vi "Do.vi"(8 "error in (no error)":errorcluster, 10 "Actor in":refnum<class "Actor.lvclass">, 11 "LogStatementMsg":refnum<class "LogStatementMsg.lvclass">) -> (0 "error out":errorcluster, 2 "Actor out":refnum<class "Actor.lvclass">)   [LabVIEW 2026, in "Lumberjack.lvlib" / "LogStatementMsg.lvclass"]
doc: "<p>(<strong>Filename</strong>: <span class=\"dnl\">Actor Framework.lvlib:Message.lvclass:Do.vi</span>)</p>\n<p>Defines what a message does when it is received by an actor. Generally, a message instructs an actor to invoke one of its methods. By default, this method does nothing. A child class must override it to define behavior.</p>"
uses:
  LogStatementMsg.lvclass
  <vilib>/ActorFramework/Actor/Actor.lvclass
  Appenders/Appender.lvclass/Appender.lvclass
  LogStatementMsg.lvclass/LogStatementMsg.ctl
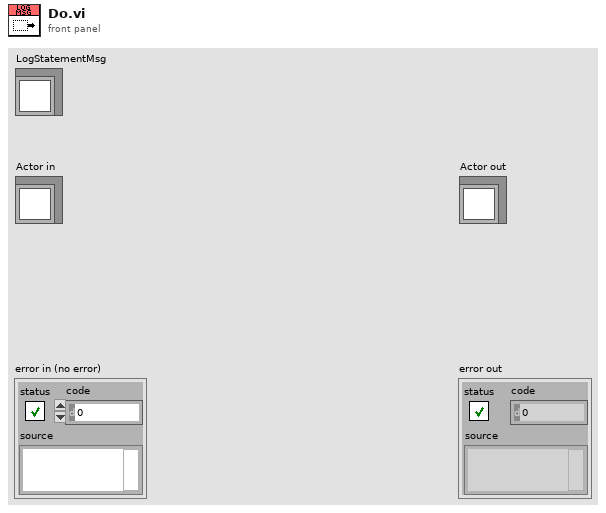
[diagram p1: front panel]
types:
  T1 = typedef "Lumberjack.lvlib/Statement.ctl" = cluster{"timestamp":timestamp, "level":T2, "sourceTag":string, "originVI":string, "message":string}
  T2 = typedef "Lumberjack.lvlib/Severity.ctl" = enum16{"OFF", "FATAL", "ERROR", "WARN", "INFO", "DEBUG", "TRACE", "ALL"}
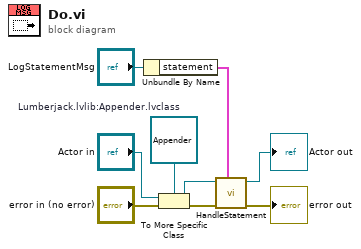
[diagram p0: block diagram]
diagram:
  w1 = refnum<class "Appender.lvclass"> refnum  # Lumberjack.lvlib:Appender.lvclass
  n1 = Unbundle By Name("LogStatementMsg") -> ("statement"=w7:T1)
  n2 = To More Specific Class(target class=w1, reference="Actor in", error in="error in (no error)") -> (specific class reference=w9:refnum<class "Appender.lvclass">, error out=w6:errorcluster)
  n3 = call "HandleStatement.vi"("Statement"=w7, "error in (no error)"=w6, "Appender in"=w9) -> ("error out"=→"error out":errorcluster, "Appender out"=→"Actor out":refnum<class "Appender.lvclass">)  [unwired: 7 in]
